vi "Broken VI.vi"   [LabVIEW 2020]
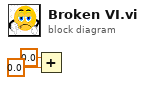
[diagram p0: block diagram]
diagram:
  n1 = Add(x=0.0, y=0.0) -> ()  [unwired: 1 out]
